vi "Cantileverbeam_experiment_data_generation.vi"() -> ()   [LabVIEW 2020]
uses:
  <vilib>/DAQmx/write.llb/DAQmx Write (Analog Wfm 1Chan NSamp).vi
  <vilib>/DAQmx/read.llb/DAQmx Read (Analog 1D Wfm NChan NSamp).vi
  <vilib>/DAQmx/create/channels.llb/DAQmx Create Channel (AO-Voltage-Basic).vi
  <vilib>/DAQmx/configure/timing.llb/DAQmx Timing (Sample Clock).vi
  <vilib>/Utility/file.llb/Read Delimited Spreadsheet (DBL).vi
  <vilib>/DAQmx/create/channels.llb/DAQmx Create Channel (AI-Voltage-Basic).vi
  <vilib>/DAQmx/create/channels.llb/DAQmx Create Channel (AI-Force-Bridge-Two-Point-Linear).vi
  <vilib>/DAQmx/create/channels.llb/DAQmx Create Channel (AI-Acceleration-Accelerometer).vi
  <vilib>/DAQmx/miscellaneous.llb/DAQmx Fill In Error Info.vi
  <resource>/objmgr/daqmx.rc
panel:
  out "Force":waveform(dbl)[](graph)
  out "Acc":waveform(dbl)[](graph)
  out "Votage in":waveform(dbl)[](graph)
  in  "Combo Box":string(combo)
  out "file location for save":path
  out "Input (Voltage out)":waveform(dbl)(graph)
  in  "file to run":path=path "C:/Users/Puja/Desktop/Labview(PC)/Input_Signal/Sine_wave_data_without_time/data1_w1_NT_1per.txt"
  in  "error in":errorcluster
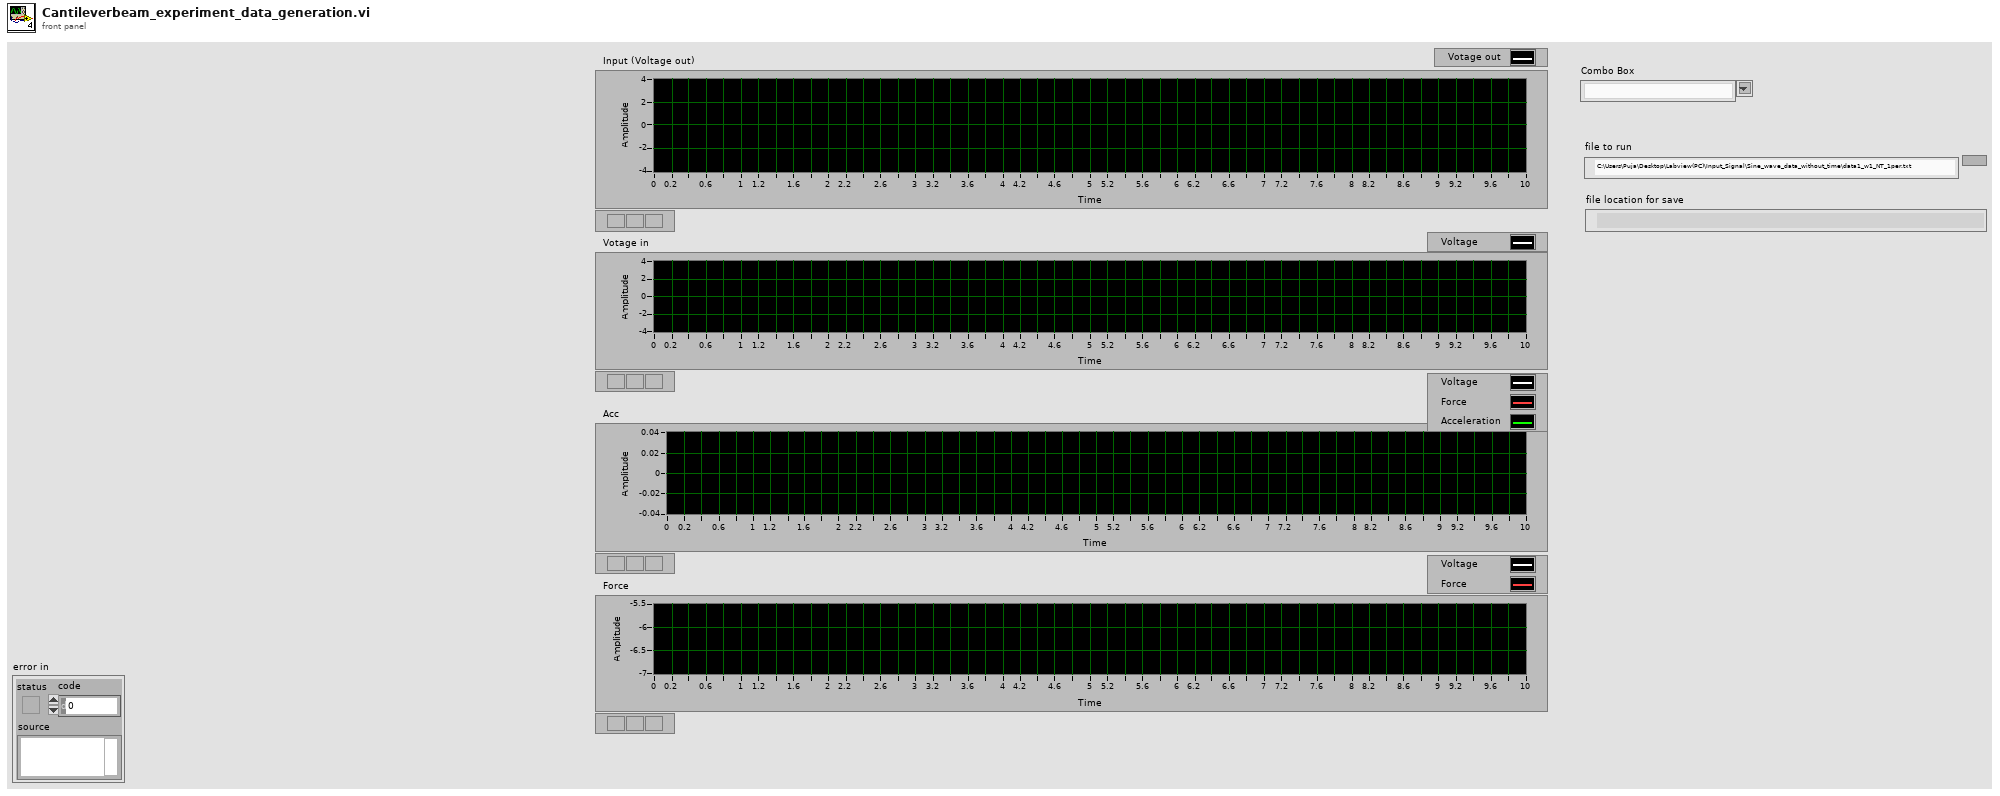
[diagram p1: front panel]
types:
  T1 = cluster{"bridge configuration":i32, "voltage excitation source":i32, "voltage excitation value":dbl, "nominal bridge resistance":dbl}
  T2 = cluster{"first electrical value":dbl, "second electrical value":dbl, "electrical units":i32, "first physical value":dbl, "second physical value":dbl, "physical units":i32}
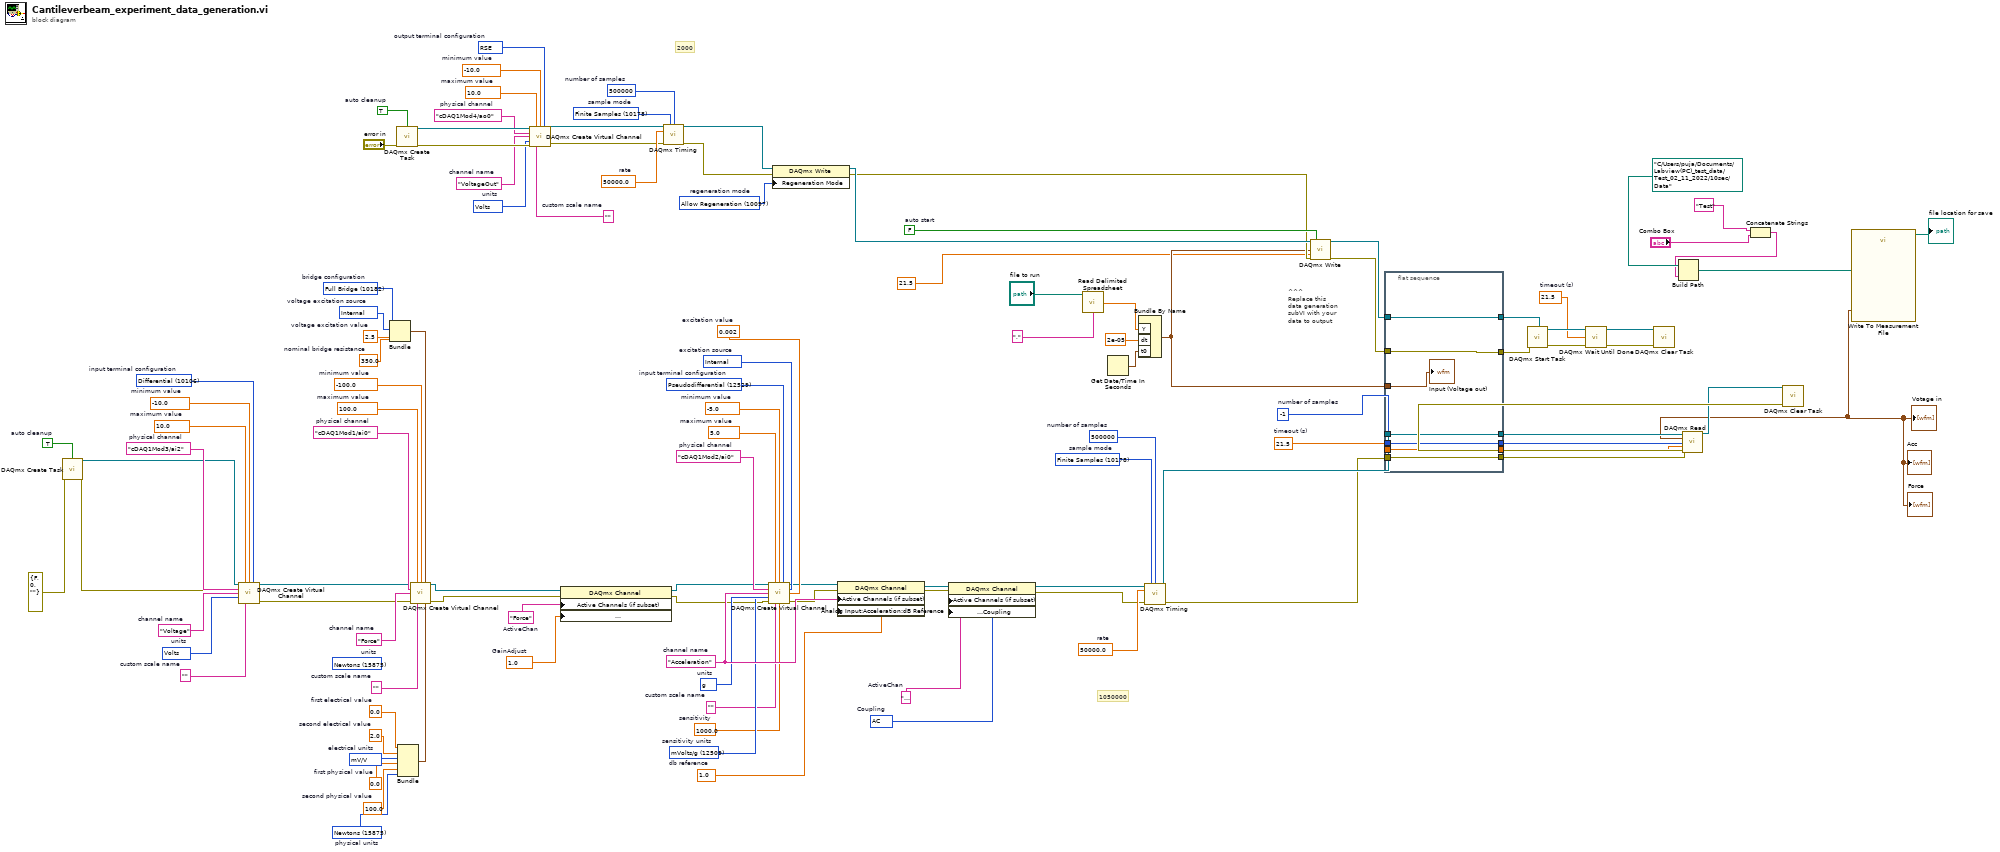
[diagram p0: block diagram]
diagram:
  w28 = 10106 items=["default"=-1, "RSE"=10083, "NRSE"=10078, "Differential"=10106, "Pseudodifferential"=12529]  # input terminal configuration
  w29 = 10348 items=["Volts"=10348, "From Custom Scale"=10065]  # units
  w30 = "Voltage"  # channel name
  w31 = ""  # custom scale name
  w32 = -10.0  # minimum value
  w33 = 10.0  # maximum value
  w34 = "cDAQ1Mod3/ai2"  # physical channel
  w35 = 1.0  # GainAdjust
  w36 = "Force"  # ActiveChan
  w37 = 15875 items=["Newtons"=15875, "Pounds"=15876, "kgf"=15877]  # physical units
  w43 = 0.0  # first electrical value
  w42 = 2.0  # second electrical value
  w41 = 15897 items=["V/V"=15896, "mV/V"=15897]  # electrical units
  w40 = 0.0  # first physical value
  w39 = 100.0  # second physical value
  w45 = 350.0  # nominal bridge resistance
  w46 = 2.5  # voltage excitation value
  w47 = 10200 items=["Internal"=10200, "External"=10167]  # voltage excitation source
  w48 = 10182 items=["Full Bridge"=10182, "Half Bridge"=10187, "Quarter Bridge"=10270]  # bridge configuration
  (unwired) 15875 items=["Newtons"=15875, "Pounds"=15876, "kgf"=15877, "From Custom Scale"=10065]  # units
  w49 = "Force"  # channel name
  w51 = ""  # custom scale name
  w52 = -100.0  # minimum value
  w53 = 100.0  # maximum value
  w54 = "cDAQ1Mod1/ai0"  # physical channel
  w81 = 10178 items=["Finite Samples"=10178, "Continuous Samples"=10123, "Hardware Timed Single Point"=12522]  # sample mode
  w80 = 500000  # number of samples
  w79 = 50000.0  # rate
  w78 = 10045 items=["AC"=10045, "DC"=10050, "GND"=10066]  # Coupling
  w77 = "Acceleration"  # ActiveChan
  w75 = 1.0  # db reference
  w73 = 10186 items=["g"=10186, "m/s^2"=12470, "From Custom Scale"=10065]  # units
  w72 = 12529 items=["default"=-1, "RSE"=10083, "NRSE"=10078, "Differential"=10106, "Pseudodifferential"=12529]  # input terminal configuration
  w71 = 10200 items=["Internal"=10200, "External"=10167, "None"=10230]  # excitation source
  w70 = 0.002  # excitation value
  w69 = 12509 items=["mVolts/g"=12509, "Volts/g"=12510]  # sensitivity units
  w68 = 1000.0  # sensitivity
  w76 = "Acceleration"  # channel name
  w66 = ""  # custom scale name
  w65 = -5.0  # minimum value
  w64 = 5.0  # maximum value
  w63 = "cDAQ1Mod2/ai0"  # physical channel
  w62 = TRUE  # auto cleanup
  w9 = 21.5  # timeout (s)
  w10 = -1  # number of samples
  w92 = 10097 items=["Allow Regeneration"=10097, "Do Not Allow Regeneration"=10158]  # regeneration mode
  w94 = 10178 items=["Finite Samples"=10178, "Continuous Samples"=10123, "Hardware Timed Single Point"=12522]  # sample mode
  w95 = 500000  # number of samples
  w96 = 50000.0  # rate
  w98 = 10083 items=["Default"=-1, "RSE"=10083, "Differential"=10106, "Pseudodifferential"=12529]  # output terminal configuration
  w99 = 10348 items=["Volts"=10348, "From Custom Scale"=10065]  # units
  w100 = "VoltageOut"  # channel name
  w101 = ""  # custom scale name
  w102 = -10.0  # minimum value
  w103 = 10.0  # maximum value
  w104 = "cDAQ1Mod4/ao0"  # physical channel
  w106 = TRUE  # auto cleanup
  w110 = 21.5  # timeout (s)
  w114 = FALSE  # auto start
  # "2000"
  # "1050000"
  # "^^^\nReplace this\ndata generation\nsubVI with your\ndata to output"
  n1 = call <vilib>:"DAQmx Create Task.vi"("auto cleanup"=w62, "error in"=errorcluster {"status"=FALSE, "code"=0, "source"=""}) -> ("task out"=w27:refnum<k21>, "error out"=w26:errorcluster)  [unwired: 12 in]
  n2 = call-poly <vilib>:"DAQmx Create Virtual Channel.vi"("task in"=w27, "maximum value"=w33, "minimum value"=w32, "input terminal configuration"=w28, "physical channels"=w34, "name to assign"=w30, "units"=w29, "error in"=w26, "custom scale name"=w31) -> ("task out"=w19:refnum<k21>, "error out"=w18:errorcluster)  [unwired: 5 in]
  n3 = Bundle("bridge configuration"=w48, "voltage excitation source"=w47, "voltage excitation value"=w46, "nominal bridge resistance"=w45) -> (w44:T1)  [unwired: 1 in]
  n4 = call <vilib>:"DAQmx Create Task.vi"("auto cleanup"=w106, "error in"="error in") -> ("task out"=w105:refnum<k21>, "error out"=w107:errorcluster)  [unwired: 12 in]
  n5 = Bundle("first electrical value"=w43, "second electrical value"=w42, "electrical units"=w41, "first physical value"=w40, "second physical value"=w39, "physical units"=w37) -> (w38:T2)  [unwired: 1 in]
  n6 = call-poly <vilib>:"DAQmx Create Virtual Channel.vi"("task in"=w19, "maximum value"=w53, "minimum value"=w52, "bridge information"=w44, "physical channels"=w54, "name to assign"=w49, "error in"=w18, "custom scale name"=w51, "scaling information"=w38) -> ("task out"=w21:refnum<k21>, "error out"=w50:errorcluster)  [unwired: 5 in]
  n7 = call-poly <vilib>:"DAQmx Create Virtual Channel.vi"("task in"=w105, "maximum value"=w103, "minimum value"=w102, "output terminal configuration"=w98, "physical channels"=w104, "name to assign"=w100, "units"=w99, "error in"=w107, "custom scale name"=w101) -> ("task out"=w97:refnum<k21>, "error out"=w16:errorcluster)  [unwired: 5 in]
  n8 = property class="DAQmx Channel"(reference=w21, error in=w50, "Active Channels (if subset)"=w36, "Analog Input:General Properties:Signal Conditioning:Bridge:Shunt Cal:Gain Adjustment"=w35) -> (reference out=w8:refnum<k21>, error out=w7:errorcluster)
  n9 = call-poly <vilib>:"DAQmx Timing.vi"("task/channels in"=w97, "sample mode"=w94, "samples per channel"=w95, "rate"=w96, "error in"=w16) -> ("task out"=w93:refnum<k21>, "error out"=w15:errorcluster)  [unwired: 9 in]
  n10 = call-poly <vilib>:"DAQmx Create Virtual Channel.vi"("task in"=w8, "maximum value"=w64, "minimum value"=w65, "input terminal configuration"=w72, "physical channels"=w63, "current excitation source"=w71, "name to assign"=w76, "current excitation value"=w70, "units"=w73, "error in"=w7, "custom scale name"=w66, "sensitivity"=w68, "sensitivity units"=w69) -> ("task out"=w67:refnum<k21>, "error out"=w74:errorcluster)  [unwired: 1 in]
  n11 = property class="DAQmx Write"(reference=w93, error in=w15, "Regeneration Mode"=w92) -> (reference out=w91:refnum<k21>, error out=w90:errorcluster)
  n12 = property class="DAQmx Channel"(reference=w67, error in=w74, "Active Channels (if subset)"=w76, "Analog Input:Acceleration:dB Reference"=w75) -> (reference out=w6:refnum<k21>, error out=w5:errorcluster)
  n13 = property class="DAQmx Channel"(reference=w6, error in=w5, "Active Channels (if subset)"=w77, "Analog Input:General Properties:Input Configuration:Coupling"=w78) -> (reference out=w12:refnum<k21>, error out=w11:errorcluster)
  n14 = call-poly <vilib>:"Read Delimited Spreadsheet.vi"("file path (dialog if empty)"="file to run", "delimiter (\\t)"=",") -> ("first row"=w2:dbl[])  [unwired: 8 in, 5 out]
  n15 = Get Date/Time In Seconds() -> (seconds since 1Jan1904=w83:timestamp)
  n16 = Bundle By Name("Y"=w2, "dt"=2e-05, "t0"=w83) -> (w14:waveform(dbl))  [unwired: 1 in]
  n17 = call-poly <vilib>:"DAQmx Timing.vi"("task/channels in"=w12, "sample mode"=w81, "samples per channel"=w80, "rate"=w79, "error in"=w11) -> ("task out"=w61:refnum<k21>, "error out"=w60:errorcluster)  [unwired: 9 in]
  n18 = call-poly <vilib>:"DAQmx Write.vi"("task/channels in"=w91, "auto start"=w114, "data"=w14, "timeout"=21.5, "error in"=w90) -> ("task out"=w89:refnum<k21>, "error out"=w87:errorcluster)  [unwired: 8 in, 1 out]
  n19 = flat-sequence {
    tunnel: w89 -> [w121]
    tunnel: w87 -> [w120]
    tunnel: w61 -> [w119]
    tunnel: w10 -> [w118]
    tunnel: w9 -> [w117]
    tunnel: w60 -> [w116]
    tunnel: w14 -> [w115]
    tunnel: [w121] -> w88
    tunnel: [w120] -> w86
    tunnel: [w119] -> w58
    tunnel: [w118] -> w57
    tunnel: [w117] -> w56
    tunnel: [w116] -> w55
    frame #0 {
      "Input (Voltage out)" <- w115
    }
  }
  n20 = call <vilib>:"DAQmx Start Task.vi"("task/channels in"=w88, "error in"=w86) -> ("task out"=w113:refnum<k21>, "error out"=w112:errorcluster)  [unwired: 12 in]
  n21 = call <vilib>:"DAQmx Wait Until Done.vi"("task/channels in"=w113, "timeout (sec)"=w110, "error in"=w112) -> ("task out"=w109:refnum<k21>, "error out"=w111:errorcluster)  [unwired: 11 in]
  n22 = call <vilib>:"DAQmx Clear Task.vi"("task in"=w109, "error in"=w111) -> ()  [unwired: 13 in, 1 out]
  n23 = call-poly <vilib>:"DAQmx Read.vi"("task/channels in"=w58, "number of samples per channel"=w57, "timeout"=w56, "error in"=w55) -> ("task out"=w3:refnum<k21>, "data"=w1:waveform(dbl)[], "error out"=w59:errorcluster)  [unwired: 9 in]
  "Votage in" <- w1
  "Acc" <- w1
  "Force" <- w1
  n24 = Concatenate Strings("Test", "Combo Box") -> (w4:string)
  n25 = Build Path(base path=path "C:/Users/puja/Documents/Labview(PC)_test_data/Test_02_11_2022/10sec/Data", name or relative path=w4) -> (appended path=w23:path)
  n26 = call <vilib>:"DAQmx Clear Task.vi"("task in"=w3, "error in"=w59) -> ()  [unwired: 13 in, 1 out]
  n27 = call "Write To Measurement File"("Signals"=w1, "Filename"=w23) -> ("Filename Out"=→"file location for save":path)  [unwired: 15 in, 2 out]
